vi "Port Config UI.vi"(8 "error in (no error)":errorcluster, 9 "Port LS":u16=5557 caption="Port for Low Speed Data", 10 "Port HS":u16=5556 caption="Port for High Speed Data", 11 "Port Rdr":u16=5555 caption="Port for Commands") -> (0 "error out":errorcluster, 1 "Canceled?":bool, 3 "Ports":T1)   [LabVIEW 2018, in "Configuration Grandmaster.lvlib" / "Cfg Grandmaster.lvclass"]
uses:
  Cfg Grandmaster.lvclass
  Common/Controls/TCP Ports.ctl
panel:
  in  "Cancel":bool
  in  "OK":bool
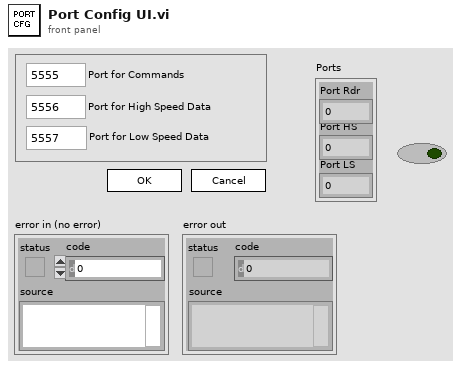
[diagram p1: front panel]
types:
  T1 = typedef "TCP Ports.ctl" = cluster{"Port Rdr":u16, "Port HS":u16, "Port LS":u16}
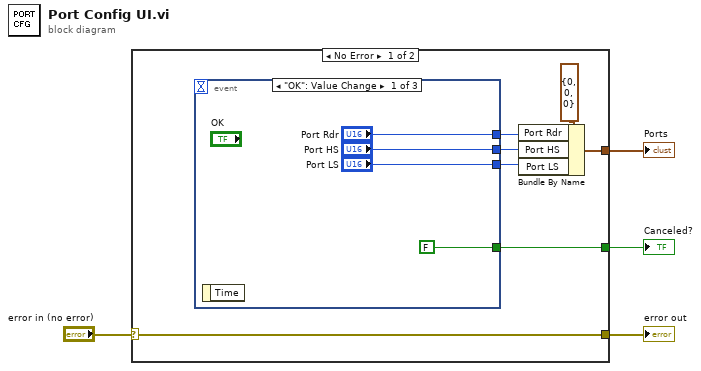
[diagram p0: block diagram]
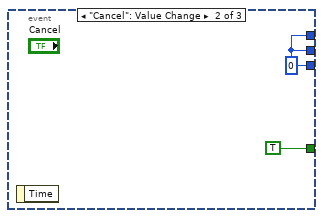
[diagram p2: hidden frame]
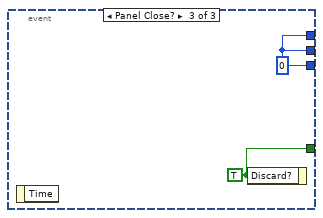
[diagram p3: hidden frame]
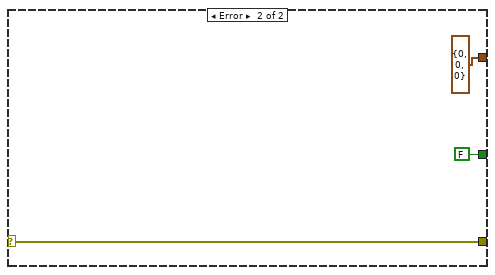
[diagram p4: hidden frame]
diagram:
  n1 = case shown="No Error" "error in (no error)" {
    selector: "error in (no error)" -> [w8 w22]
    tunnel: [w8 w22] -> w3
    tunnel: [w7 T1 {"Port Rdr"=0, "Port HS"=0, "Port LS"=0} ("output cluster")] -> w2
    tunnel: [w6 FALSE ("Discard?")] -> w1
    frame No Error {
      n2 = event shown="[0] \"OK\": Value Change" {
        selector: _ -> [_ _ _]
        dyn-events: _ -> [_ _ _]
        timeout: _ -> [_ _ _]
        tunnel: ["Port LS" w16 w18] -> w9
        tunnel: ["Port HS" w16 w18] -> w10
        tunnel: [FALSE TRUE w19] -> w6
        tunnel: ["Port Rdr" w16 w18] -> w5
        event "OK": Value Change {
          n3 = event-data() -> ()  [unwired: 1 in, 1 out]
        }
        event "Cancel": Value Change {
          w16 = u16 0 ("Port LS")
          n4 = event-data() -> ()  [unwired: 1 in, 1 out]
        }
        event Panel Close? {
          w18 = u16 0 ("Port LS")
          w19 = TRUE ("Discard?")
          n5 = event-data() -> ()  [unwired: 1 in, 1 out]
          n6 = event-data("Discard?"=w19) -> ()  [unwired: 1 in, 1 out]
        }
      }
      n7 = Bundle By Name(cluster=T1 {"Port Rdr"=0, "Port HS"=0, "Port LS"=0} ("output cluster"), "Port Rdr"=w5, "Port HS"=w10, "Port LS"=w9) -> (w7:T1)
    }
    frame Error {
    }
  }
  "error out" <- w3
  "Ports" <- w2
  "Canceled?" <- w1
